vi "Module Name--constant.vi"() -> (3 "Module Name":string)   [LabVIEW 2024, in "MoneyControl.lvlib"]
doc: "Return the name of the module that owns this VI. \n_____\nBased on DQMH Dev Tools: Project Template 7.1.0.1503."
uses:
  MoneyControl.lvlib
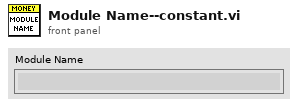
[diagram p1: front panel]
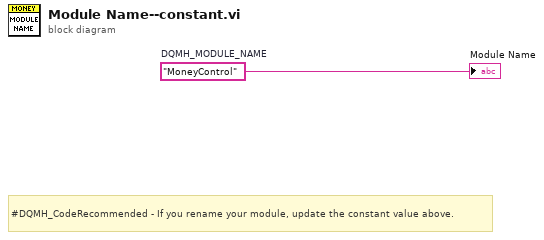
[diagram p0: block diagram]
diagram:
  w1 = "MoneyControl"  # DQMH_MODULE_NAME
  # "#DQMH_CodeRecommended - If you rename your module, update the constant value above."
  "Module Name" <- w1
